vi "HB_GetFirmwareVersion.vi"(8 "error in (no error)":errorcluster, 11 "HBDeviceRef":T1) -> (0 "error IO":errorcluster, 1 "Firmware Version":string, 2 "Version Byte Array":u8[](array[numeric]), 3 "HBDeviceRef":T1)   [LabVIEW 2016]
doc: "Returns the version of the firmware on the Huskie Board formatted as a byte array and a version string. The version string is formatted as: major.minor.fix.test which also corresponds to the byte array."
uses:
  <vilib>/Rock Robotics/WPI/SerialPort/WPI_SerialPortRef.ctl
  <vilib>/Utility/error.llb/Error Cluster From Error Code.vi
  <vilib>/ErrorRing/Error Ring.xnode
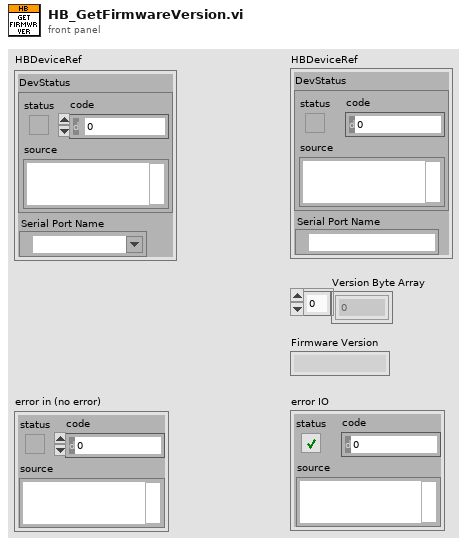
[diagram p1: front panel]
types:
  T1 = typedef "WPI_SerialPortRef.ctl" = cluster{"DevStatus":errorcluster, "Serial Port Name":refnum<visa-resource-name>}
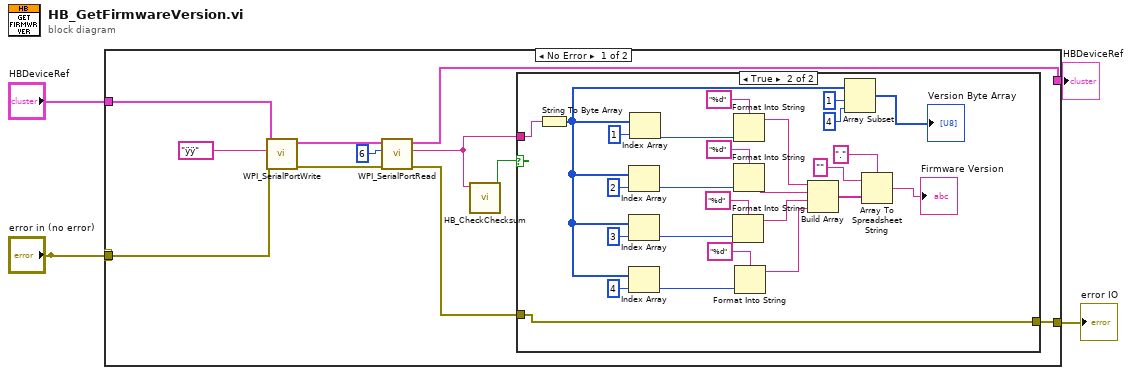
[diagram p0: block diagram]
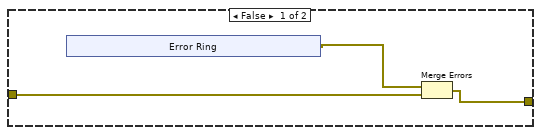
[diagram p2: hidden frame]
diagram:
  n1 = case shown="No Error" "error in (no error)" {
    selector: "error in (no error)" -> [_ w49]
    tunnel: "HBDeviceRef" -> [w12 w50]
    tunnel: "error in (no error)" -> [w11 _]
    tunnel: [w9 w50] -> w1
    tunnel: [w5 w49] -> w2
    frame No Error {
      n2 = call <vilib>:"WPI_SerialPortWrite.vi"("error in (no error)"=w11, "Buffer"="ÿÿ", "SerialPortRef"=w12) -> ("error out"=w13:errorcluster, "SerialPortRef"=w14:T1)  [unwired: 6 in, 1 out]
      n3 = call <vilib>:"WPI_SerialPortRead.vi"("error in (no error)"=w13, "Num Bytes to Read"=u32 6, "SerialPortRef"=w14) -> ("error out"=w6:errorcluster, "Buffer"=w7:string, "SerialPortRef"=w9:T1)  [unwired: 6 in]
      n4 = call "HB_CheckChecksum.vi"("String"=w7) -> ("Checksum Matches"=w8:bool)  [unwired: 9 in, 1 out]
      n5 = case shown="True" w8 {
        tunnel: w7 -> [_ w26]
        tunnel: w6 -> [w18 w25]
        tunnel: [w17 w25] -> w5
        frame False {
          n6 = xnode "Error Ring"() -> ("error out"=w16:errorcluster)
          n7 = Merge Errors(w16, w18) -> (w17:errorcluster)
        }
        frame True {
          n8 = String To Byte Array(string=w26) -> (unsigned byte array=w30:u8[])
          n9 = Index Array(array=w30, index=2) -> (element=w39:u8)
          n10 = Index Array(array=w30, index=3) -> (element=w38:u8)
          n11 = Index Array(array=w30, index=4) -> (element=w37:u8)
          n12 = Index Array(array=w30, index=1) -> (element=w44:u8)
          n13 = Format Into String(format string="%d", w38) -> (resulting string=w34:string)  [unwired: 2 in, 1 out]
          n14 = Format Into String(format string="%d", w44) -> (resulting string=w36:string)  [unwired: 2 in, 1 out]
          n15 = Format Into String(format string="%d", w39) -> (resulting string=w35:string)  [unwired: 2 in, 1 out]
          n16 = Format Into String(format string="%d", w37) -> (resulting string=w33:string)  [unwired: 2 in, 1 out]
          n17 = Build Array(w36, w35, w34, w33) -> (w24:string[])
          n18 = Array Subset(array=w30, index=1, length=4) -> (→"Version Byte Array":u8[])
          n19 = Array To Spreadsheet String(delimiter (Tab)=".", array=w24, 3:"" ("format string")) -> (spreadsheet string=→"Firmware Version":string)
        }
      }
    }
    frame Error {
    }
  }
  "HBDeviceRef" <- w1
  "error IO" <- w2
